vi "HandleObservationSync_002.vi"(8 "error in (no error)":errorcluster, 11 "S4GUI in":refnum<class "S4GUI.lvclass">) -> (0 "error out":errorcluster, 3 "S4GUI out":refnum<class "S4GUI.lvclass">)   [LabVIEW 2018, in "S4GUI.lvclass"] (continued)
          n221 = call "Read Instrument.lvclass.vi"("error in (no error)"=w570, "S4ACS_GUI in"=w571) -> ("error out"=w541:errorcluster, "Instrument.lvclass"=w542:refnum<class "Instrument.lvclass">, "S4ACS_GUI out"=w572:refnum<class "S4GUI.lvclass">)  [unwired: 7 in]
          n222 = disable-structure shown="Enabled" {
            disable-tunnel: w542 -> [w576 w589]
            disable-tunnel: w541 -> [w575 w588]
            disable-tunnel: [w574 w589] -> w540
            disable-tunnel: [w573 w588] -> w539
            frame Disabled {
              n223 = call "Read WPROT.vi"("error in (no error)"=w575, "Instrument in"=w576) -> ("error out"=w579:errorcluster, "Opt_Selector.lvclass"=w580:refnum<class "Opt_Selector.lvclass">, "Instrument out"=w586:refnum<class "Instrument.lvclass">)  [unwired: 7 in]
              n224 = call-dynamic "Read State Machine.vi"("error in (no error)"=w579, "Device in"=w580) -> ("error out"=w582:errorcluster, "State Machine.lvclass"=w584:refnum<class "State Machine.lvclass">, "Device out"=w581:refnum<class "Opt_Selector.lvclass">)  [unwired: 7 in]
              n225 = call "Next State.vi"("error in (no error)"=w582, "New_State"=30, "State Machine in"=w584) -> ("error out"=w578:errorcluster, "State Machine out"=w577:refnum<class "State Machine.lvclass">)  [unwired: 7 in]
              n226 = call-dynamic "Write State Machine.vi"("error in (no error)"=w578, "State Machine.lvclass"=w577, "Device in"=w581) -> ("error out"=w585:errorcluster, "Device out"=w587:refnum<class "Opt_Selector.lvclass">)  [unwired: 7 in]
              n227 = call "Write WPROT.vi"("error in (no error)"=w585, "Opt_Selector.lvclass"=w587, "Instrument in"=w586) -> ("error out"=w573:errorcluster, "Instrument out"=w574:refnum<class "Instrument.lvclass">)  [unwired: 7 in]
            }
            frame Enabled {
              # "depois do homing no WPSEL, o homing do WPROT é feito automaticamente pelo ICS"
            }
          }
          n228 = call "Read ASEL.vi"("error in (no error)"=w539, "Instrument in"=w540) -> ("error out"=w556:errorcluster, "Opt_Selector.lvclass"=w557:refnum<class "Opt_Selector.lvclass">, "Instrument out"=w563:refnum<class "Instrument.lvclass">)  [unwired: 7 in]
          n229 = call-dynamic "Read State Machine.vi"("error in (no error)"=w556, "Device in"=w557) -> ("error out"=w559:errorcluster, "State Machine.lvclass"=w561:refnum<class "State Machine.lvclass">, "Device out"=w558:refnum<class "Opt_Selector.lvclass">)  [unwired: 7 in]
          n230 = call "Next State.vi"("error in (no error)"=w559, "New_State"=30, "State Machine in"=w561) -> ("error out"=w555:errorcluster, "State Machine out"=w554:refnum<class "State Machine.lvclass">)  [unwired: 7 in]
          n231 = call-dynamic "Write State Machine.vi"("error in (no error)"=w555, "State Machine.lvclass"=w554, "Device in"=w558) -> ("error out"=w562:errorcluster, "Device out"=w564:refnum<class "Opt_Selector.lvclass">)  [unwired: 7 in]
          n232 = Increment(x=w565) -> (x+1=w567:u32)
          n233 = call "Write ASEL.vi"("error in (no error)"=w562, "Opt_Selector.lvclass"=w564, "Instrument in"=w563) -> ("error out"=w537:errorcluster, "Instrument out"=w538:refnum<class "Instrument.lvclass">)  [unwired: 7 in]
          n234 = call "Read GMIR.vi"("error in (no error)"=w537, "Instrument in"=w538) -> ("error out"=w545:errorcluster, "Opt_Continuous.lvclass"=w546:refnum<class "Opt_Continuous.lvclass">, "Instrument out"=w552:refnum<class "Instrument.lvclass">)  [unwired: 7 in]
          n235 = call-dynamic "Read State Machine.vi"("error in (no error)"=w545, "Device in"=w546) -> ("error out"=w548:errorcluster, "State Machine.lvclass"=w550:refnum<class "State Machine.lvclass">, "Device out"=w547:refnum<class "Opt_Continuous.lvclass">)  [unwired: 7 in]
          n236 = call "Next State.vi"("error in (no error)"=w548, "New_State"=30, "State Machine in"=w550) -> ("error out"=w544:errorcluster, "State Machine out"=w543:refnum<class "State Machine.lvclass">)  [unwired: 7 in]
          n237 = call-dynamic "Write State Machine.vi"("error in (no error)"=w544, "State Machine.lvclass"=w543, "Device in"=w547) -> ("error out"=w551:errorcluster, "Device out"=w553:refnum<class "Opt_Continuous.lvclass">)  [unwired: 7 in]
          n238 = call "Write GMIR.vi"("error in (no error)"=w551, "Opt_Continuous.lvclass"=w553, "Instrument in"=w552) -> ("error out"=w536:errorcluster, "Instrument out"=w535:refnum<class "Instrument.lvclass">)  [unwired: 7 in]
          n239 = call "Write Instrument.lvclass.vi"("error in (no error)"=w536, "Instrument.lvclass"=w535, "S4ACS_GUI in"=w572) -> ("error out"=w569:errorcluster, "S4ACS_GUI out"=w568:refnum<class "S4GUI.lvclass">)  [unwired: 7 in]
          n240 = Bundle By Name(cluster=w568, "Obs_state"=w567) -> (w566:refnum<class "S4GUI.lvclass">)
        }
        frame 223 {
          # "Espera terminar o homing de WPROT,ASEL e GFOC\nantes de seguir para o próximo estado."
          n241 = call "Read Instrument.lvclass.vi"("error in (no error)"=w614, "S4ACS_GUI in"=w615) -> ("error out"=w600:errorcluster, "Instrument.lvclass"=w601:refnum<class "Instrument.lvclass">, "S4ACS_GUI out"=w609:refnum<class "S4GUI.lvclass">)  [unwired: 7 in]
          n242 = call "Read ASEL.vi"("error in (no error)"=w600, "Instrument in"=w601) -> ("error out"=w605:errorcluster, "Opt_Selector.lvclass"=w591:refnum<class "Opt_Selector.lvclass">)  [unwired: 7 in, 1 out]
          n243 = call "Read GMIR.vi"("error in (no error)"=w600, "Instrument in"=w601) -> ("error out"=w602:errorcluster, "Opt_Continuous.lvclass"=w590:refnum<class "Opt_Continuous.lvclass">)  [unwired: 7 in, 1 out]
          n244 = disable-structure shown="Enabled" {
            disable-tunnel: [w619 w625] -> w608
            disable-tunnel: w601 -> [w618 _]
            disable-tunnel: w600 -> [w617 w625]
            disable-tunnel: [w616 0 ("State")] -> w599
            frame Disabled {
              n245 = call "Read WPROT.vi"("error in (no error)"=w617, "Instrument in"=w618) -> ("error out"=w621:errorcluster, "Opt_Selector.lvclass"=w620:refnum<class "Opt_Selector.lvclass">)  [unwired: 7 in, 1 out]
              n246 = call-dynamic "Read State Machine.vi"("error in (no error)"=w621, "Device in"=w620) -> ("error out"=w622:errorcluster, "State Machine.lvclass"=w623:refnum<class "State Machine.lvclass">)  [unwired: 7 in, 1 out]
              n247 = call-dynamic "Read State.vi"("error in (no error)"=w622, "State Machine in"=w623) -> ("error out"=w619:errorcluster, "State"=w616:i32)  [unwired: 7 in, 1 out]
            }
            frame Enabled {
            }
          }
          n248 = call-dynamic "Read State Machine.vi"("error in (no error)"=w605, "Device in"=w591) -> ("error out"=w606:errorcluster, "State Machine.lvclass"=w607:refnum<class "State Machine.lvclass">)  [unwired: 7 in, 1 out]
          n249 = call-dynamic "Read State Machine.vi"("error in (no error)"=w602, "Device in"=w590) -> ("error out"=w603:errorcluster, "State Machine.lvclass"=w604:refnum<class "State Machine.lvclass">)  [unwired: 7 in, 1 out]
          n250 = Increment(x=w611) -> (x+1=w610:u32)
          n251 = call-dynamic "Read State.vi"("error in (no error)"=w606, "State Machine in"=w607) -> ("error out"=w594:errorcluster, "State"=w598:i32)  [unwired: 7 in, 1 out]
          n252 = call-dynamic "Read State.vi"("error in (no error)"=w603, "State Machine in"=w604) -> ("error out"=w593:errorcluster, "State"=w597:i32)  [unwired: 7 in, 1 out]
          n253 = Compound Arithmetic op=ADD(w599, w598, w597) -> (w596:i32)
          n254 = Equal To 0?(x=w596) -> (x = 0?=w595:bool)
          n255 = Merge Errors(w608, w594, w593) -> (w592:errorcluster)
          n256 = Select(t=w610, s=w595, f=w611) -> (s? t:f=w612:u32)
          n257 = Bundle By Name(cluster=w609, "Obs_state"=w612) -> (w613:refnum<class "S4GUI.lvclass">)
        }
        frame 224 {
          # "40 x 0.25 = 10s"
          # "40 x 0.25 = 10s"
          # "40 x 0.25 = 10s"
          # "Manda WPSEL para OFF, CALW para OFF e ASEL para OFF"
          n258 = call "Read Instrument.lvclass.vi"("error in (no error)"=w699, "S4ACS_GUI in"=w700) -> ("error out"=w685:errorcluster, "Instrument.lvclass"=w686:refnum<class "Instrument.lvclass">, "S4ACS_GUI out"=w701:refnum<class "S4GUI.lvclass">)  [unwired: 7 in]
          n259 = call "Read WPSEL.vi"("error in (no error)"=w685, "Instrument in"=w686) -> ("error out"=w681:errorcluster, "Opt_Selector.lvclass"=w680:refnum<class "Opt_Selector.lvclass">, "Instrument out"=w693:refnum<class "Instrument.lvclass">)  [unwired: 7 in]
          n260 = call "Write target.vi"("error in (no error)"=w681, "target"=80.0, "Optics in"=w680) -> ("error out"=w684:errorcluster, "Optics out"=w679:refnum<class "Opt_Selector.lvclass">)  [unwired: 7 in]
          n261 = call "Write target name.vi"("error in (no error)"=w684, "target name"="OFF", "Optics in"=w679) -> ("error out"=w677:errorcluster, "Optics out"=w678:refnum<class "Opt_Selector.lvclass">)  [unwired: 7 in]
          n262 = call-dynamic "Read State Machine.vi"("error in (no error)"=w677, "Device in"=w678) -> ("error out"=w688:errorcluster, "State Machine.lvclass"=w690:refnum<class "State Machine.lvclass">, "Device out"=w687:refnum<class "Opt_Selector.lvclass">)  [unwired: 7 in]
          n263 = call "Next State.vi"("error in (no error)"=w688, "New_State"=1, "State Machine in"=w690) -> ("error out"=w638:errorcluster, "State Machine out"=w640:refnum<class "State Machine.lvclass">)  [unwired: 7 in]
          n264 = call-dynamic "Write Timer.vi"("error in (no error)"=w638, "Timer"=u32 40, "State Machine in"=w640) -> ("error out"=w637:errorcluster, "State Machine out"=w639:refnum<class "State Machine.lvclass">)  [unwired: 7 in]
          n265 = call-dynamic "Write State Machine.vi"("error in (no error)"=w637, "State Machine.lvclass"=w639, "Device in"=w687) -> ("error out"=w692:errorcluster, "Device out"=w694:refnum<class "Opt_Selector.lvclass">)  [unwired: 7 in]
          n266 = Increment(x=w691) -> (x+1=w696:u32)
          n267 = call "Write WPSEL.vi"("error in (no error)"=w692, "Opt_Selector.lvclass"=w694, "Instrument in"=w693) -> ("error out"=w652:errorcluster, "Instrument out"=w651:refnum<class "Instrument.lvclass">)  [unwired: 7 in]
          n268 = call "Read CALW.vi"("error in (no error)"=w652, "Instrument in"=w651) -> ("error out"=w668:errorcluster, "Opt_Selector.lvclass"=w650:refnum<class "Opt_Selector.lvclass">, "Instrument out"=w648:refnum<class "Instrument.lvclass">)  [unwired: 7 in]
          n269 = call "Write target.vi"("error in (no error)"=w668, "target"=0.0, "Optics in"=w650) -> ("error out"=w671:errorcluster, "Optics out"=w667:refnum<class "Opt_Selector.lvclass">)  [unwired: 7 in]
          n270 = call "Write target name.vi"("error in (no error)"=w671, "target name"="OFF", "Optics in"=w667) -> ("error out"=w665:errorcluster, "Optics out"=w666:refnum<class "Opt_Selector.lvclass">)  [unwired: 7 in]
          n271 = call-dynamic "Read State Machine.vi"("error in (no error)"=w665, "Device in"=w666) -> ("error out"=w673:errorcluster, "State Machine.lvclass"=w675:refnum<class "State Machine.lvclass">, "Device out"=w672:refnum<class "Opt_Selector.lvclass">)  [unwired: 7 in]
          n272 = call "Next State.vi"("error in (no error)"=w673, "New_State"=1, "State Machine in"=w675) -> ("error out"=w634:errorcluster, "State Machine out"=w635:refnum<class "State Machine.lvclass">)  [unwired: 7 in]
          n273 = call-dynamic "Write Timer.vi"("error in (no error)"=w634, "Timer"=u32 40, "State Machine in"=w635) -> ("error out"=w633:errorcluster, "State Machine out"=w632:refnum<class "State Machine.lvclass">)  [unwired: 7 in]
          n274 = call-dynamic "Write State Machine.vi"("error in (no error)"=w633, "State Machine.lvclass"=w632, "Device in"=w672) -> ("error out"=w676:errorcluster, "Device out"=w649:refnum<class "Opt_Selector.lvclass">)  [unwired: 7 in]
          n275 = call "Write CALW.vi"("error in (no error)"=w676, "Opt_Selector.lvclass"=w649, "Instrument in"=w648) -> ("error out"=w647:errorcluster, "Instrument out"=w646:refnum<class "Instrument.lvclass">)  [unwired: 7 in]
          n276 = call "Read ASEL.vi"("error in (no error)"=w647, "Instrument in"=w646) -> ("error out"=w656:errorcluster, "Opt_Selector.lvclass"=w645:refnum<class "Opt_Selector.lvclass">, "Instrument out"=w643:refnum<class "Instrument.lvclass">)  [unwired: 7 in]
          n277 = call "Write target.vi"("error in (no error)"=w656, "target"=0.0, "Optics in"=w645) -> ("error out"=w659:errorcluster, "Optics out"=w655:refnum<class "Opt_Selector.lvclass">)  [unwired: 7 in]
          n278 = call "Write target name.vi"("error in (no error)"=w659, "target name"="OFF", "Optics in"=w655) -> ("error out"=w653:errorcluster, "Optics out"=w654:refnum<class "Opt_Selector.lvclass">)  [unwired: 7 in]
          n279 = call-dynamic "Read State Machine.vi"("error in (no error)"=w653, "Device in"=w654) -> ("error out"=w661:errorcluster, "State Machine.lvclass"=w663:refnum<class "State Machine.lvclass">, "Device out"=w660:refnum<class "Opt_Selector.lvclass">)  [unwired: 7 in]
          n280 = call "Next State.vi"("error in (no error)"=w661, "New_State"=1, "State Machine in"=w663) -> ("error out"=w628:errorcluster, "State Machine out"=w629:refnum<class "State Machine.lvclass">)  [unwired: 7 in]
          n281 = call-dynamic "Write Timer.vi"("error in (no error)"=w628, "Timer"=u32 40, "State Machine in"=w629) -> ("error out"=w627:errorcluster, "State Machine out"=w626:refnum<class "State Machine.lvclass">)  [unwired: 7 in]
          n282 = call-dynamic "Write State Machine.vi"("error in (no error)"=w627, "State Machine.lvclass"=w626, "Device in"=w660) -> ("error out"=w664:errorcluster, "Device out"=w644:refnum<class "Opt_Selector.lvclass">)  [unwired: 7 in]
          n283 = call "Write ASEL.vi"("error in (no error)"=w664, "Opt_Selector.lvclass"=w644, "Instrument in"=w643) -> ("error out"=w641:errorcluster, "Instrument out"=w642:refnum<class "Instrument.lvclass">)  [unwired: 7 in]
          n284 = call "Write Instrument.lvclass.vi"("error in (no error)"=w641, "Instrument.lvclass"=w642, "S4ACS_GUI in"=w701) -> ("error out"=w698:errorcluster, "S4ACS_GUI out"=w697:refnum<class "S4GUI.lvclass">)  [unwired: 7 in]
          n285 = Bundle By Name(cluster=w697, "Obs_state"=w696) -> (w695:refnum<class "S4GUI.lvclass">)
        }
        frame 225 {
          # "Espera terminar o movimento de WPSEL, ASEL e CALW para CLEAR."
          n286 = call "Read Instrument.lvclass.vi"("error in (no error)"=w730, "S4ACS_GUI in"=w731) -> ("error out"=w713:errorcluster, "Instrument.lvclass"=w714:refnum<class "Instrument.lvclass">, "S4ACS_GUI out"=w722:refnum<class "S4GUI.lvclass">)  [unwired: 7 in]
          n287 = call "Read ASEL.vi"("error in (no error)"=w713, "Instrument in"=w714) -> ("error out"=w718:errorcluster, "Opt_Selector.lvclass"=w704:refnum<class "Opt_Selector.lvclass">)  [unwired: 7 in, 1 out]
          n288 = call "Read CALW.vi"("error in (no error)"=w713, "Instrument in"=w714) -> ("error out"=w715:errorcluster, "Opt_Selector.lvclass"=w703:refnum<class "Opt_Selector.lvclass">)  [unwired: 7 in, 1 out]
          n289 = call "Read WPSEL.vi"("error in (no error)"=w713, "Instrument in"=w714) -> ("error out"=w727:errorcluster, "Opt_Selector.lvclass"=w726:refnum<class "Opt_Selector.lvclass">)  [unwired: 7 in, 1 out]
          n290 = call-dynamic "Read State Machine.vi"("error in (no error)"=w715, "Device in"=w703) -> ("error out"=w716:errorcluster, "State Machine.lvclass"=w717:refnum<class "State Machine.lvclass">)  [unwired: 7 in, 1 out]
          n291 = call-dynamic "Read State Machine.vi"("error in (no error)"=w718, "Device in"=w704) -> ("error out"=w719:errorcluster, "State Machine.lvclass"=w720:refnum<class "State Machine.lvclass">)  [unwired: 7 in, 1 out]
          n292 = call-dynamic "Read State Machine.vi"("error in (no error)"=w727, "Device in"=w726) -> ("error out"=w728:errorcluster, "State Machine.lvclass"=w729:refnum<class "State Machine.lvclass">)  [unwired: 7 in, 1 out]
          n293 = call-dynamic "Read State.vi"("error in (no error)"=w719, "State Machine in"=w720) -> ("error out"=w707:errorcluster, "State"=w711:i32)  [unwired: 7 in, 1 out]
          n294 = call-dynamic "Read State.vi"("error in (no error)"=w716, "State Machine in"=w717) -> ("error out"=w706:errorcluster, "State"=w710:i32)  [unwired: 7 in, 1 out]
          n295 = call-dynamic "Read State.vi"("error in (no error)"=w728, "State Machine in"=w729) -> ("error out"=w721:errorcluster, "State"=w712:i32)  [unwired: 7 in, 1 out]
          n296 = Compound Arithmetic op=ADD(w712, w711, w710) -> (w709:i32)
          n297 = Equal To 0?(x=w709) -> (x = 0?=w708:bool)
          n298 = Merge Errors(w721, w707, w706) -> (w705:errorcluster)
          n299 = Select(t=u32 0, s=w708, f=w723) -> (s? t:f=w724:u32)
          n300 = Bundle By Name(cluster=w722, "Obs_state"=w724) -> (w725:refnum<class "S4GUI.lvclass">)
        }
        frame 230 {
          # "PARK:\nWPSEL = OFF\n(WPROT=NA)\nCALW=SHUTTER\nASEL=OFF"
          n301 = call "Read Instrument.lvclass.vi"("error in (no error)"=w799, "S4ACS_GUI in"=w800) -> ("error out"=w792:errorcluster, "Instrument.lvclass"=w793:refnum<class "Instrument.lvclass">, "S4ACS_GUI out"=w734:refnum<class "S4GUI.lvclass">)  [unwired: 7 in]
          n302 = call "Read WPSEL.vi"("error in (no error)"=w792, "Instrument in"=w793) -> ("error out"=w755:errorcluster, "Opt_Selector.lvclass"=w758:refnum<class "Opt_Selector.lvclass">, "Instrument out"=w788:refnum<class "Instrument.lvclass">)  [unwired: 7 in]
          n303 = call "Write target name.vi"("error in (no error)"=w755, "target name"="OFF", "Optics in"=w758) -> ("error out"=w754:errorcluster, "Optics out"=w757:refnum<class "Opt_Selector.lvclass">)  [unwired: 7 in]
          n304 = call "Write target.vi"("error in (no error)"=w754, "target"=80.0, "Optics in"=w757) -> ("error out"=w753:errorcluster, "Optics out"=w756:refnum<class "Opt_Selector.lvclass">)  [unwired: 7 in]
          n305 = call-dynamic "Read State Machine.vi"("error in (no error)"=w753, "Device in"=w756) -> ("error out"=w784:errorcluster, "State Machine.lvclass"=w786:refnum<class "State Machine.lvclass">, "Device out"=w783:refnum<class "Opt_Selector.lvclass">)  [unwired: 7 in]
          n306 = call "Next State.vi"("error in (no error)"=w784, "New_State"=1, "State Machine in"=w786) -> ("error out"=w763:errorcluster, "State Machine out"=w764:refnum<class "State Machine.lvclass">)  [unwired: 7 in]
          n307 = call-dynamic "Write State Machine.vi"("error in (no error)"=w763, "State Machine.lvclass"=w764, "Device in"=w783) -> ("error out"=w787:errorcluster, "Device out"=w789:refnum<class "Opt_Selector.lvclass">)  [unwired: 7 in]
          n308 = Increment(x=w794) -> (x+1=w796:u32)
          n309 = call "Write WPSEL.vi"("error in (no error)"=w787, "Opt_Selector.lvclass"=w789, "Instrument in"=w788) -> ("error out"=w767:errorcluster, "Instrument out"=w768:refnum<class "Instrument.lvclass">)  [unwired: 7 in]
          n310 = call "Read CALW.vi"("error in (no error)"=w767, "Instrument in"=w768) -> ("error out"=w747:errorcluster, "Opt_Selector.lvclass"=w746:refnum<class "Opt_Selector.lvclass">, "Instrument out"=w781:refnum<class "Instrument.lvclass">)  [unwired: 7 in]
          n311 = call "Write target name.vi"("error in (no error)"=w747, "target name"="SHUTTER", "Optics in"=w746) -> ("error out"=w750:errorcluster, "Optics out"=w745:refnum<class "Opt_Selector.lvclass">)  [unwired: 7 in]
          n312 = call "Write target.vi"("error in (no error)"=w750, "target"=216.0, "Optics in"=w745) -> ("error out"=w743:errorcluster, "Optics out"=w744:refnum<class "Opt_Selector.lvclass">)  [unwired: 7 in]
          n313 = call-dynamic "Read State Machine.vi"("error in (no error)"=w743, "Device in"=w744) -> ("error out"=w777:errorcluster, "State Machine.lvclass"=w779:refnum<class "State Machine.lvclass">, "Device out"=w776:refnum<class "Opt_Selector.lvclass">)  [unwired: 7 in]
          n314 = call "Next State.vi"("error in (no error)"=w777, "New_State"=1, "State Machine in"=w779) -> ("error out"=w761:errorcluster, "State Machine out"=w762:refnum<class "State Machine.lvclass">)  [unwired: 7 in]
          n315 = call-dynamic "Write State Machine.vi"("error in (no error)"=w761, "State Machine.lvclass"=w762, "Device in"=w776) -> ("error out"=w780:errorcluster, "Device out"=w782:refnum<class "Opt_Selector.lvclass">)  [unwired: 7 in]
          n316 = call "Write CALW.vi"("error in (no error)"=w780, "Opt_Selector.lvclass"=w782, "Instrument in"=w781) -> ("error out"=w765:errorcluster, "Instrument out"=w766:refnum<class "Instrument.lvclass">)  [unwired: 7 in]
          n317 = call "Read ASEL.vi"("error in (no error)"=w765, "Instrument in"=w766) -> ("error out"=w736:errorcluster, "Opt_Selector.lvclass"=w739:refnum<class "Opt_Selector.lvclass">, "Instrument out"=w774:refnum<class "Instrument.lvclass">)  [unwired: 7 in]
          n318 = call "Write target name.vi"("error in (no error)"=w736, "target name"="OFF", "Optics in"=w739) -> ("error out"=w742:errorcluster, "Optics out"=w738:refnum<class "Opt_Selector.lvclass">)  [unwired: 7 in]
          n319 = call "Write target.vi"("error in (no error)"=w742, "target"=0.0, "Optics in"=w738) -> ("error out"=w735:errorcluster, "Optics out"=w737:refnum<class "Opt_Selector.lvclass">)  [unwired: 7 in]
          n320 = call-dynamic "Read State Machine.vi"("error in (no error)"=w735, "Device in"=w737) -> ("error out"=w770:errorcluster, "State Machine.lvclass"=w772:refnum<class "State Machine.lvclass">, "Device out"=w769:refnum<class "Opt_Selector.lvclass">)  [unwired: 7 in]
          n321 = call "Next State.vi"("error in (no error)"=w770, "New_State"=1, "State Machine in"=w772) -> ("error out"=w759:errorcluster, "State Machine out"=w760:refnum<class "State Machine.lvclass">)  [unwired: 7 in]
          n322 = call-dynamic "Write State Machine.vi"("error in (no error)"=w759, "State Machine.lvclass"=w760, "Device in"=w769) -> ("error out"=w773:errorcluster, "Device out"=w775:refnum<class "Opt_Selector.lvclass">)  [unwired: 7 in]
          n323 = call "Write ASEL.vi"("error in (no error)"=w773, "Opt_Selector.lvclass"=w775, "Instrument in"=w774) -> ("error out"=w791:errorcluster, "Instrument out"=w790:refnum<class "Instrument.lvclass">)  [unwired: 7 in]
          n324 = Bundle By Name(cluster=w734, "Error Msg"="Parking in progress. Wait....") -> (w733:refnum<class "S4GUI.lvclass">)
          n325 = call "Write Instrument.lvclass.vi"("error in (no error)"=w791, "Instrument.lvclass"=w790, "S4ACS_GUI in"=w733) -> ("error out"=w798:errorcluster, "S4ACS_GUI out"=w797:refnum<class "S4GUI.lvclass">)  [unwired: 7 in]
          n326 = Bundle By Name(cluster=w797, "Obs_state"=w796) -> (w795:refnum<class "S4GUI.lvclass">)
        }
        frame 231 {
          # "Espera terminar o parking de WPSEL,CALW e ASEL\nantes de encerrar aplicacao (exit=True)."
          n327 = call "Read Instrument.lvclass.vi"("error in (no error)"=w829, "S4ACS_GUI in"=w830) -> ("error out"=w811:errorcluster, "Instrument.lvclass"=w812:refnum<class "Instrument.lvclass">, "S4ACS_GUI out"=w820:refnum<class "S4GUI.lvclass">)  [unwired: 7 in]
          n328 = call "Read CALW.vi"("error in (no error)"=w811, "Instrument in"=w812) -> ("error out"=w816:errorcluster, "Opt_Selector.lvclass"=w802:refnum<class "Opt_Selector.lvclass">)  [unwired: 7 in, 1 out]
          n329 = call "Read ASEL.vi"("error in (no error)"=w811, "Instrument in"=w812) -> ("error out"=w813:errorcluster, "Opt_Selector.lvclass"=w801:refnum<class "Opt_Selector.lvclass">)  [unwired: 7 in, 1 out]
          n330 = call "Read WPSEL.vi"("error in (no error)"=w811, "Instrument in"=w812) -> ("error out"=w826:errorcluster, "Opt_Selector.lvclass"=w825:refnum<class "Opt_Selector.lvclass">)  [unwired: 7 in, 1 out]
          n331 = call-dynamic "Read State Machine.vi"("error in (no error)"=w816, "Device in"=w802) -> ("error out"=w817:errorcluster, "State Machine.lvclass"=w818:refnum<class "State Machine.lvclass">)  [unwired: 7 in, 1 out]
          n332 = call-dynamic "Read State Machine.vi"("error in (no error)"=w813, "Device in"=w801) -> ("error out"=w814:errorcluster, "State Machine.lvclass"=w815:refnum<class "State Machine.lvclass">)  [unwired: 7 in, 1 out]
          n333 = call-dynamic "Read State Machine.vi"("error in (no error)"=w826, "Device in"=w825) -> ("error out"=w827:errorcluster, "State Machine.lvclass"=w828:refnum<class "State Machine.lvclass">)  [unwired: 7 in, 1 out]
          n334 = Increment(x=w822) -> (x+1=w821:u32)
          n335 = call-dynamic "Read State.vi"("error in (no error)"=w817, "State Machine in"=w818) -> ("error out"=w805:errorcluster, "State"=w809:i32)  [unwired: 7 in, 1 out]
          n336 = call-dynamic "Read State.vi"("error in (no error)"=w814, "State Machine in"=w815) -> ("error out"=w804:errorcluster, "State"=w808:i32)  [unwired: 7 in, 1 out]
          n337 = call-dynamic "Read State.vi"("error in (no error)"=w827, "State Machine in"=w828) -> ("error out"=w819:errorcluster, "State"=w810:i32)  [unwired: 7 in, 1 out]
          n338 = Compound Arithmetic op=ADD(w810, w809, w808) -> (w807:i32)
          n339 = Equal To 0?(x=w807) -> (x = 0?=w806:bool)
          n340 = Merge Errors(w819, w805, w804) -> (w803:errorcluster)
          n341 = Select(t=w821, s=w806, f=w822) -> (s? t:f=w823:u32)
          n342 = Bundle By Name(cluster=w820, "Obs_state"=w823) -> (w824:refnum<class "S4GUI.lvclass">)
        }
        frame 232 {
          n343 = Increment(x=w832) -> (x+1=w831:u32)
          n344 = Tick Count (ms)() -> (millisecond timer value=w833:u32)
          n345 = local write "time1"(w833) -> ()
          n346 = Bundle By Name(cluster=w836, "Obs_state"=w831) -> (w834:refnum<class "S4GUI.lvclass">)
        }
        frame 233 {
          # "Aguarda 1s para atualização do painel da GUI antes de encerrar..."
          n347 = local read "time1"() -> (w840:u32)
          n348 = Tick Count (ms)() -> (millisecond timer value=w841:u32)
          n349 = Subtract(x=w841, y=w840) -> (x-y=w839:u32)
          n350 = Greater?(x=w839, y=u32 1000) -> (0:w837:bool)
          n351 = case shown="True" w837 {
            tunnel: w843 -> [w847 w849]
            tunnel: [w847 w848] -> w842
            frame False {
            }
            frame True {
              n352 = Increment(x=w849) -> (x+1=w848:u32)
            }
          }
          n353 = Bundle By Name(cluster=w846, "Obs_state"=w842) -> (w844:refnum<class "S4GUI.lvclass">)
        }
        frame 234 {
          n354 = Bundle By Name(cluster=w854, "Obs_state"=u32 0, "exit"=TRUE) -> (w852:refnum<class "S4GUI.lvclass">)
        }
        frame 251 {
          n355 = flat-sequence {
            tunnel: w903 -> [w1058]
            tunnel: [w1058] -> w902
            frame #0 {
              n356 = Tick Count (ms)() -> (millisecond timer value=→"time3":u32)
            }
          }
          n357 = call-dynamic "Read AcquisitionA.vi"("error in (no error)"=w902, "S4ACS_GUI in"=w920) -> ("error out"=w887:errorcluster, "Acquisition.lvclass"=w885:refnum<class "Acquisition.lvclass">, "S4ACS_GUI out"=w922:refnum<class "S4GUI.lvclass">)  [unwired: 7 in]
          n358 = call-dynamic "Read enabled.vi"("error in (no error)"=w887, "Server in"=w885) -> ("error out"=w886:errorcluster, "enabled"=w882:bool, "Server out"=w884:refnum<class "Acquisition.lvclass">)  [unwired: 7 in]
          n359 = call "Read connection.vi"("error in (no error)"=w886, "Server in"=w884) -> ("error out"=w918:errorcluster, "connection"=w888:bool, "Server out"=w917:refnum<class "Acquisition.lvclass">)  [unwired: 7 in]
          n360 = And(x=w888, y=w882) -> (x .and. y?=w883:bool)
          n361 = case shown="True" w883 {
            tunnel: [w1038 w1057] -> w923
            tunnel: [w1037 w1056] -> w921
            tunnel: w918 -> [w1037 w1055]
            tunnel: w917 -> [w1038 w1054]
            tunnel: w882 -> [w1034 _]
            tunnel: [w1033 u32 0] -> w881
            frame False {
              n362 = Select(t=u32 1, s=w1034, f=u32 0) -> (s? t:f=w1033:u32)
            }
            frame True {
              # "configura o canal,\nmas não dispara\na exposicao."
              n363 = call-dynamic "Read Channel.vi"("error in (no error)"=w1055, "Acquisition in"=w1054) -> ("error out"=w1044:errorcluster, "Channel.lvclass"=w1046:refnum<class "Channel.lvclass">, "Acquisition out"=w1053:refnum<class "Acquisition.lvclass">)  [unwired: 7 in]
              n364 = call-dynamic "Write expose.vi"("error in (no error)"=w1044, "expose"=FALSE, "Channel in"=w1046) -> ("error out"=w1043:errorcluster, "Channel out"=w1045:refnum<class "Channel.lvclass">)  [unwired: 7 in]
              n365 = call-dynamic "Read State Machine.vi"("error in (no error)"=w1043, "Device in"=w1045) -> ("error out"=w1050:errorcluster, "State Machine.lvclass"=w1052:refnum<class "State Machine.lvclass">, "Device out"=w1048:refnum<class "Channel.lvclass">)  [unwired: 7 in]
              n366 = call "Next State.vi"("error in (no error)"=w1050, "New_State"=1, "State Machine in"=w1052) -> ("error out"=w1040:errorcluster, "State Machine out"=w1041:refnum<class "State Machine.lvclass">)  [unwired: 7 in]
              n367 = call-dynamic "Write State Machine.vi"("error in (no error)"=w1040, "State Machine.lvclass"=w1041, "Device in"=w1048) -> ("error out"=w1047:errorcluster, "Device out"=w1049:refnum<class "Channel.lvclass">)  [unwired: 7 in]
              n368 = call-dynamic "Write Channel.vi"("error in (no error)"=w1047, "Channel.lvclass"=w1049, "Acquisition in"=w1053) -> ("error out"=w1056:errorcluster, "Acquisition out"=w1057:refnum<class "Acquisition.lvclass">)  [unwired: 7 in]
            }
          }
          n369 = call-dynamic "Write AcquisitionA.vi"("error in (no error)"=w921, "Acquisition.lvclass"=w923, "S4ACS_GUI in"=w922) -> ("error out"=w913:errorcluster, "S4ACS_GUI out"=w912:refnum<class "S4GUI.lvclass">)  [unwired: 7 in]
          n370 = call "Read AcquisitionB.vi"("error in (no error)"=w913, "S4ACS_GUI in"=w912) -> ("error out"=w871:errorcluster, "Acquisition.lvclass"=w873:refnum<class "Acquisition.lvclass">, "S4ACS_GUI out"=w914:refnum<class "S4GUI.lvclass">)  [unwired: 7 in]
          n371 = call-dynamic "Read enabled.vi"("error in (no error)"=w871, "Server in"=w873) -> ("error out"=w870:errorcluster, "enabled"=w855:bool, "Server out"=w872:refnum<class "Acquisition.lvclass">)  [unwired: 7 in]
          n372 = call "Read connection.vi"("error in (no error)"=w870, "Server in"=w872) -> ("error out"=w899:errorcluster, "connection"=w874:bool, "Server out"=w900:refnum<class "Acquisition.lvclass">)  [unwired: 7 in]
          n373 = And(x=w874, y=w855) -> (x .and. y?=w875:bool)
          n374 = case shown="True" w875 {
            tunnel: [w1013 w1032] -> w898
            tunnel: [w1012 w1031] -> w897
            tunnel: w899 -> [w1012 w1030]
            tunnel: w900 -> [w1013 w1029]
            tunnel: [w1009 u32 0 ("f")] -> w878
            tunnel: w855 -> [w1008 _]
            frame False {
              n375 = Select(t=u32 2, s=w1008, f=u32 0) -> (s? t:f=w1009:u32)
            }
            frame True {
              # "configura o canal,\nmas não dispara\na exposicao."
              n376 = call-dynamic "Read Channel.vi"("error in (no error)"=w1030, "Acquisition in"=w1029) -> ("error out"=w1019:errorcluster, "Channel.lvclass"=w1021:refnum<class "Channel.lvclass">, "Acquisition out"=w1028:refnum<class "Acquisition.lvclass">)  [unwired: 7 in]
              n377 = call-dynamic "Write expose.vi"("error in (no error)"=w1019, "expose"=FALSE, "Channel in"=w1021) -> ("error out"=w1018:errorcluster, "Channel out"=w1020:refnum<class "Channel.lvclass">)  [unwired: 7 in]
              n378 = call-dynamic "Read State Machine.vi"("error in (no error)"=w1018, "Device in"=w1020) -> ("error out"=w1025:errorcluster, "State Machine.lvclass"=w1027:refnum<class "State Machine.lvclass">, "Device out"=w1023:refnum<class "Channel.lvclass">)  [unwired: 7 in]
              n379 = call "Next State.vi"("error in (no error)"=w1025, "New_State"=1, "State Machine in"=w1027) -> ("error out"=w1015:errorcluster, "State Machine out"=w1016:refnum<class "State Machine.lvclass">)  [unwired: 7 in]
              n380 = call-dynamic "Write State Machine.vi"("error in (no error)"=w1015, "State Machine.lvclass"=w1016, "Device in"=w1023) -> ("error out"=w1022:errorcluster, "Device out"=w1024:refnum<class "Channel.lvclass">)  [unwired: 7 in]
              n381 = call-dynamic "Write Channel.vi"("error in (no error)"=w1022, "Channel.lvclass"=w1024, "Acquisition in"=w1028) -> ("error out"=w1031:errorcluster, "Acquisition out"=w1032:refnum<class "Acquisition.lvclass">)  [unwired: 7 in]
            }
          }
          n382 = call "Write AcquisitionB.vi"("error in (no error)"=w897, "Acquisition.lvclass"=w898, "S4ACS_GUI in"=w914) -> ("error out"=w909:errorcluster, "S4ACS_GUI out"=w908:refnum<class "S4GUI.lvclass">)  [unwired: 7 in]
          n383 = call-dynamic "Read AcquisitionC.vi"("error in (no error)"=w909, "S4ACS_GUI in"=w908) -> ("error out"=w867:errorcluster, "Acquisition.lvclass"=w869:refnum<class "Acquisition.lvclass">, "S4ACS_GUI out"=w911:refnum<class "S4GUI.lvclass">)  [unwired: 7 in]
          n384 = call-dynamic "Read enabled.vi"("error in (no error)"=w867, "Server in"=w869) -> ("error out"=w866:errorcluster, "enabled"=w856:bool, "Server out"=w868:refnum<class "Acquisition.lvclass">)  [unwired: 7 in]
          n385 = call "Read connection.vi"("error in (no error)"=w866, "Server in"=w868) -> ("error out"=w895:errorcluster, "connection"=w865:bool, "Server out"=w896:refnum<class "Acquisition.lvclass">)  [unwired: 7 in]
          n386 = And(x=w865, y=w856) -> (x .and. y?=w864:bool)
          n387 = case shown="True" w864 {
            tunnel: [w988 w1007] -> w894
            tunnel: [w987 w1006] -> w893
            tunnel: w895 -> [w987 w1005]
            tunnel: w896 -> [w988 w1004]
            tunnel: [w984 u32 0 ("f")] -> w877
            tunnel: w856 -> [w983 _]
            frame False {
              n388 = Select(t=u32 4, s=w983, f=u32 0) -> (s? t:f=w984:u32)
            }
            frame True {
              # "configura o canal,\nmas não dispara\na exposicao."
              n389 = call-dynamic "Read Channel.vi"("error in (no error)"=w1005, "Acquisition in"=w1004) -> ("error out"=w994:errorcluster, "Channel.lvclass"=w996:refnum<class "Channel.lvclass">, "Acquisition out"=w1003:refnum<class "Acquisition.lvclass">)  [unwired: 7 in]
              n390 = call-dynamic "Write expose.vi"("error in (no error)"=w994, "expose"=FALSE, "Channel in"=w996) -> ("error out"=w993:errorcluster, "Channel out"=w995:refnum<class "Channel.lvclass">)  [unwired: 7 in]
              n391 = call-dynamic "Read State Machine.vi"("error in (no error)"=w993, "Device in"=w995) -> ("error out"=w1000:errorcluster, "State Machine.lvclass"=w1002:refnum<class "State Machine.lvclass">, "Device out"=w998:refnum<class "Channel.lvclass">)  [unwired: 7 in]
              n392 = call "Next State.vi"("error in (no error)"=w1000, "New_State"=1, "State Machine in"=w1002) -> ("error out"=w990:errorcluster, "State Machine out"=w991:refnum<class "State Machine.lvclass">)  [unwired: 7 in]
              n393 = call-dynamic "Write State Machine.vi"("error in (no error)"=w990, "State Machine.lvclass"=w991, "Device in"=w998) -> ("error out"=w997:errorcluster, "Device out"=w999:refnum<class "Channel.lvclass">)  [unwired: 7 in]
              n394 = call-dynamic "Write Channel.vi"("error in (no error)"=w997, "Channel.lvclass"=w999, "Acquisition in"=w1003) -> ("error out"=w1006:errorcluster, "Acquisition out"=w1007:refnum<class "Acquisition.lvclass">)  [unwired: 7 in]
            }
          }
          n395 = call-dynamic "Write AcquisitionC.vi"("error in (no error)"=w893, "Acquisition.lvclass"=w894, "S4ACS_GUI in"=w911) -> ("error out"=w907:errorcluster, "S4ACS_GUI out"=w906:refnum<class "S4GUI.lvclass">)  [unwired: 7 in]
          n396 = call-dynamic "Read AcquisitionD.vi"("error in (no error)"=w907, "S4ACS_GUI in"=w906) -> ("error out"=w861:errorcluster, "Acquisition.lvclass"=w863:refnum<class "Acquisition.lvclass">, "S4ACS_GUI out"=w910:refnum<class "S4GUI.lvclass">)  [unwired: 7 in]
          n397 = call-dynamic "Read enabled.vi"("error in (no error)"=w861, "Server in"=w863) -> ("error out"=w860:errorcluster, "enabled"=w857:bool, "Server out"=w862:refnum<class "Acquisition.lvclass">)  [unwired: 7 in]
          n398 = call "Read connection.vi"("error in (no error)"=w860, "Server in"=w862) -> ("error out"=w891:errorcluster, "connection"=w859:bool, "Server out"=w892:refnum<class "Acquisition.lvclass">)  [unwired: 7 in]
          n399 = And(x=w859, y=w857) -> (x .and. y?=w858:bool)
          n400 = case shown="True" w858 {
            tunnel: [w963 w982] -> w890
            tunnel: [w962 w981] -> w889
            tunnel: w891 -> [w962 w980]
            tunnel: w892 -> [w963 w979]
            tunnel: [w959 u32 0 ("f")] -> w876
            tunnel: w857 -> [w958 _]
            frame False {
              n401 = Select(t=u32 8, s=w958, f=u32 0) -> (s? t:f=w959:u32)
            }
            frame True {
              # "configura o canal,\nmas não dispara\na exposicao."
              n402 = call-dynamic "Read Channel.vi"("error in (no error)"=w980, "Acquisition in"=w979) -> ("error out"=w969:errorcluster, "Channel.lvclass"=w971:refnum<class "Channel.lvclass">, "Acquisition out"=w978:refnum<class "Acquisition.lvclass">)  [unwired: 7 in]
              n403 = call-dynamic "Write expose.vi"("error in (no error)"=w969, "expose"=FALSE, "Channel in"=w971) -> ("error out"=w968:errorcluster, "Channel out"=w970:refnum<class "Channel.lvclass">)  [unwired: 7 in]
              n404 = call-dynamic "Read State Machine.vi"("error in (no error)"=w968, "Device in"=w970) -> ("error out"=w975:errorcluster, "State Machine.lvclass"=w977:refnum<class "State Machine.lvclass">, "Device out"=w973:refnum<class "Channel.lvclass">)  [unwired: 7 in]
              n405 = call "Next State.vi"("error in (no error)"=w975, "New_State"=1, "State Machine in"=w977) -> ("error out"=w965:errorcluster, "State Machine out"=w966:refnum<class "State Machine.lvclass">)  [unwired: 7 in]
              n406 = call-dynamic "Write State Machine.vi"("error in (no error)"=w965, "State Machine.lvclass"=w966, "Device in"=w973) -> ("error out"=w972:errorcluster, "Device out"=w974:refnum<class "Channel.lvclass">)  [unwired: 7 in]
              n407 = call-dynamic "Write Channel.vi"("error in (no error)"=w972, "Channel.lvclass"=w974, "Acquisition in"=w978) -> ("error out"=w981:errorcluster, "Acquisition out"=w982:refnum<class "Acquisition.lvclass">)  [unwired: 7 in]
            }
          }
          n408 = call-dynamic "Write AcquisitionD.vi"("error in (no error)"=w889, "Acquisition.lvclass"=w890, "S4ACS_GUI in"=w910) -> ("error out"=w905:errorcluster, "S4ACS_GUI out"=w904:refnum<class "S4GUI.lvclass">)  [unwired: 7 in]
          n409 = Compound Arithmetic op=ADD(w881, w878, w877, w876) -> (w880:u32)
          n410 = case shown="0, Default" w880 {
            tunnel: w916 -> [w927 _ _ _ _ _ _ _ _ _ _ _ _ _ _ _]
            tunnel: [w926 u32 1 ("Obs_state") u32 1 ("Obs_state") u32 1 ("Obs_state") u32 1 ("Obs_state") u32 1 ("Obs_state") u32 1 ("Obs_state") u32 1 ("Obs_state") u32 1 ("Obs_state") u32 1 ("Obs_state") u32 1 ("Obs_state") u32 1 ("Obs_state") u32 1 ("Obs_state") u32 1 ("Obs_state") u32 1 ("Obs_state") u32 1 ("Obs_state")] -> w915
            tunnel: ["" ("Error Msg") "ERROR: Lost channel 1 connection... - HandleObservationSync.vi state 251" ("Error Msg") "ERROR: Lost channel 2 connection...- HandleObservationSync.vi state 251" ("Error Msg") "ERROR: Lost channels 1 and 2 connection...- HandleObservationSync.vi state 251" ("Error Msg") "ERROR: Lost channel 3 connection...- HandleObservationSync.vi state 251" ("Error Msg") "ERROR: Lost channels 1 and  3 connection...- HandleObservationSync.vi state 251" ("Error Msg") "ERROR:  Lost channels 2 and  3 connection...- HandleObservationSync.vi state 251" ("Error Msg") "ERROR:  Lost channels 1, 2 and  3 connection...- HandleObservationSync.vi state 251" ("Error Msg") "ERROR: Lost channel 4 connection...- HandleObservationSync.vi state 251" ("Error Msg") "ERROR:  Lost channels 1 and 4 connection...- HandleObservationSync.vi state 251" ("Error Msg") "ERROR:  Lost channels 2 and 4 connection...- HandleObservationSync.vi state 251" ("Error Msg") "ERROR: Lost channels 1, 2 and 4 connection...- HandleObservationSync.vi state 251" ("Error Msg") "ERROR: Lost channels 3 and 4 connection...- HandleObservationSync.vi state 251" ("Error Msg") "ERROR: Lost channels 1, 3 and 4 connection...- HandleObservationSync.vi state 251" ("Error Msg") "ERROR: Lost channels 2, 3 and 4 connection...- HandleObservationSync.vi state 251" ("Error Msg") "ERROR: Lost channels 1, 2, 3 and 4 connection...- HandleObservationSync.vi state 251" ("Error Msg")] -> w879
            frame 0, Default {
              n411 = Tick Count (ms)() -> (millisecond timer value=→"time307":u32)
              n412 = Increment(x=w927) -> (x+1=w926:u32)
            }
            frame 1 {
            }
            frame 2 {
            }
            frame 3 {
            }
            frame 4 {
            }
            frame 5 {
            }
            frame 6 {
            }
            frame 7 {
            }
            frame 8 {
            }
            frame 9 {
            }
            frame 10 {
            }
            frame 11 {
            }
            frame 12 {
            }
            frame 13 {
            }
            frame 14 {
            }
            frame 15 {
            }
          }
          n413 = Bundle By Name(cluster=w904, "Obs_state"=w915, "cyclesDone"=u32 0, "Error Msg"=w879) -> (w919:refnum<class "S4GUI.lvclass">)
        }
        frame 252 {
          w1081 = 38 ("x")
          w1084 = 28 ("x")
          # "Se algum canal foi pra 38: Texp inválido \npara a configuração do CCD."
          # "Se algum canal foi pra 28: ERRO na inicialização."
          # "Espera terminar a execução da preparação\ndos 4 canais antes de ir ao proximo passo \nda Observação."
          n414 = flat-sequence {
            tunnel: w1113 -> [w1250]
            tunnel: [w1250] -> w1112
            frame #0 {
              n415 = Tick Count (ms)() -> (millisecond timer value=→"time4":u32)
            }
          }
          n416 = call-dynamic "Read AcquisitionA.vi"("error in (no error)"=w1112, "S4ACS_GUI in"=w1122) -> ("error out"=w1110:errorcluster, "Acquisition.lvclass"=w1111:refnum<class "Acquisition.lvclass">, "S4ACS_GUI out"=w1124:refnum<class "S4GUI.lvclass">)  [unwired: 7 in]
          n417 = call "Read connection.vi"("error in (no error)"=w1110, "Server in"=w1111) -> ("error out"=w1108:errorcluster, "connection"=w1107:bool, "Server out"=w1109:refnum<class "Acquisition.lvclass">)  [unwired: 7 in]
          n418 = case shown="True" w1107 {
            tunnel: w1109 -> [w1233 w1249]
            tunnel: w1108 -> [w1232 w1248]
            tunnel: [w1233 w1246] -> w1125
            tunnel: [w1232 w1245] -> w1123
            tunnel: [0 ("State") w1235] -> w1080
            frame False {
            }
            frame True {
              n419 = call-dynamic "Read Channel.vi"("error in (no error)"=w1248, "Acquisition in"=w1249) -> ("error out"=w1244:errorcluster, "Channel.lvclass"=w1243:refnum<class "Channel.lvclass">, "Acquisition out"=w1247:refnum<class "Acquisition.lvclass">)  [unwired: 7 in]
              n420 = call-dynamic "Read State Machine.vi"("error in (no error)"=w1244, "Device in"=w1243) -> ("error out"=w1237:errorcluster, "State Machine.lvclass"=w1239:refnum<class "State Machine.lvclass">, "Device out"=w1241:refnum<class "Channel.lvclass">)  [unwired: 7 in]
              n421 = call-dynamic "Read State.vi"("error in (no error)"=w1237, "State Machine in"=w1239) -> ("error out"=w1236:errorcluster, "State"=w1235:i32, "State Machine out"=w1238:refnum<class "State Machine.lvclass">)  [unwired: 7 in]
              n422 = call-dynamic "Write State Machine.vi"("error in (no error)"=w1236, "State Machine.lvclass"=w1238, "Device in"=w1241) -> ("error out"=w1240:errorcluster, "Device out"=w1242:refnum<class "Channel.lvclass">)  [unwired: 7 in]
              n423 = call-dynamic "Write Channel.vi"("error in (no error)"=w1240, "Channel.lvclass"=w1242, "Acquisition in"=w1247) -> ("error out"=w1245:errorcluster, "Acquisition out"=w1246:refnum<class "Acquisition.lvclass">)  [unwired: 7 in]
            }
          }
          n424 = call-dynamic "Write AcquisitionA.vi"("error in (no error)"=w1123, "Acquisition.lvclass"=w1125, "S4ACS_GUI in"=w1124) -> ("error out"=w1119:errorcluster, "S4ACS_GUI out"=w1118:refnum<class "S4GUI.lvclass">)  [unwired: 7 in]
          n425 = call "Read AcquisitionB.vi"("error in (no error)"=w1119, "S4ACS_GUI in"=w1118) -> ("error out"=w1102:errorcluster, "Acquisition.lvclass"=w1105:refnum<class "Acquisition.lvclass">, "S4ACS_GUI out"=w1106:refnum<class "S4GUI.lvclass">)  [unwired: 7 in]
          n426 = call "Read connection.vi"("error in (no error)"=w1102, "Server in"=w1105) -> ("error out"=w1101:errorcluster, "connection"=w1103:bool, "Server out"=w1104:refnum<class "Acquisition.lvclass">)  [unwired: 7 in]
          n427 = case shown="True" w1103 {
            tunnel: w1104 -> [w1215 w1231]
            tunnel: w1101 -> [w1214 w1230]
            tunnel: [w1215 w1228] -> w1100
            tunnel: [w1214 w1227] -> w1099
            tunnel: [0 ("State") w1217] -> w1079
            frame False {
            }
            frame True {
              n428 = call-dynamic "Read Channel.vi"("error in (no error)"=w1230, "Acquisition in"=w1231) -> ("error out"=w1226:errorcluster, "Channel.lvclass"=w1225:refnum<class "Channel.lvclass">, "Acquisition out"=w1229:refnum<class "Acquisition.lvclass">)  [unwired: 7 in]
              n429 = call-dynamic "Read State Machine.vi"("error in (no error)"=w1226, "Device in"=w1225) -> ("error out"=w1219:errorcluster, "State Machine.lvclass"=w1221:refnum<class "State Machine.lvclass">, "Device out"=w1223:refnum<class "Channel.lvclass">)  [unwired: 7 in]
              n430 = call-dynamic "Read State.vi"("error in (no error)"=w1219, "State Machine in"=w1221) -> ("error out"=w1218:errorcluster, "State"=w1217:i32, "State Machine out"=w1220:refnum<class "State Machine.lvclass">)  [unwired: 7 in]
              n431 = call-dynamic "Write State Machine.vi"("error in (no error)"=w1218, "State Machine.lvclass"=w1220, "Device in"=w1223) -> ("error out"=w1222:errorcluster, "Device out"=w1224:refnum<class "Channel.lvclass">)  [unwired: 7 in]
              n432 = call-dynamic "Write Channel.vi"("error in (no error)"=w1222, "Channel.lvclass"=w1224, "Acquisition in"=w1229) -> ("error out"=w1227:errorcluster, "Acquisition out"=w1228:refnum<class "Acquisition.lvclass">)  [unwired: 7 in]
            }
          }
          n433 = call "Write AcquisitionB.vi"("error in (no error)"=w1099, "Acquisition.lvclass"=w1100, "S4ACS_GUI in"=w1106) -> ("error out"=w1117:errorcluster, "S4ACS_GUI out"=w1116:refnum<class "S4GUI.lvclass">)  [unwired: 7 in]
          n434 = call-dynamic "Read AcquisitionC.vi"("error in (no error)"=w1117, "S4ACS_GUI in"=w1116) -> ("error out"=w1097:errorcluster, "Acquisition.lvclass"=w1098:refnum<class "Acquisition.lvclass">, "S4ACS_GUI out"=w1121:refnum<class "S4GUI.lvclass">)  [unwired: 7 in]
          n435 = call "Read connection.vi"("error in (no error)"=w1097, "Server in"=w1098) -> ("error out"=w1096:errorcluster, "connection"=w1094:bool, "Server out"=w1095:refnum<class "Acquisition.lvclass">)  [unwired: 7 in]
          n436 = case shown="True" w1094 {
            tunnel: w1095 -> [w1197 w1213]
            tunnel: w1096 -> [w1196 w1212]
            tunnel: [w1197 w1210] -> w1093
            tunnel: [w1196 w1209] -> w1092
            tunnel: [0 ("State") w1199] -> w1078
            frame False {
            }
            frame True {
              n437 = call-dynamic "Read Channel.vi"("error in (no error)"=w1212, "Acquisition in"=w1213) -> ("error out"=w1208:errorcluster, "Channel.lvclass"=w1207:refnum<class "Channel.lvclass">, "Acquisition out"=w1211:refnum<class "Acquisition.lvclass">)  [unwired: 7 in]
              n438 = call-dynamic "Read State Machine.vi"("error in (no error)"=w1208, "Device in"=w1207) -> ("error out"=w1201:errorcluster, "State Machine.lvclass"=w1203:refnum<class "State Machine.lvclass">, "Device out"=w1205:refnum<class "Channel.lvclass">)  [unwired: 7 in]
              n439 = call-dynamic "Read State.vi"("error in (no error)"=w1201, "State Machine in"=w1203) -> ("error out"=w1200:errorcluster, "State"=w1199:i32, "State Machine out"=w1202:refnum<class "State Machine.lvclass">)  [unwired: 7 in]
              n440 = call-dynamic "Write State Machine.vi"("error in (no error)"=w1200, "State Machine.lvclass"=w1202, "Device in"=w1205) -> ("error out"=w1204:errorcluster, "Device out"=w1206:refnum<class "Channel.lvclass">)  [unwired: 7 in]
              n441 = call-dynamic "Write Channel.vi"("error in (no error)"=w1204, "Channel.lvclass"=w1206, "Acquisition in"=w1211) -> ("error out"=w1209:errorcluster, "Acquisition out"=w1210:refnum<class "Acquisition.lvclass">)  [unwired: 7 in]
            }
          }
          n442 = call-dynamic "Write AcquisitionC.vi"("error in (no error)"=w1092, "Acquisition.lvclass"=w1093, "S4ACS_GUI in"=w1121) -> ("error out"=w1115:errorcluster, "S4ACS_GUI out"=w1114:refnum<class "S4GUI.lvclass">)  [unwired: 7 in]
          n443 = call-dynamic "Read AcquisitionD.vi"("error in (no error)"=w1115, "S4ACS_GUI in"=w1114) -> ("error out"=w1089:errorcluster, "Acquisition.lvclass"=w1091:refnum<class "Acquisition.lvclass">, "S4ACS_GUI out"=w1120:refnum<class "S4GUI.lvclass">)  [unwired: 7 in]
          n444 = call "Read connection.vi"("error in (no error)"=w1089, "Server in"=w1091) -> ("error out"=w1088:errorcluster, "connection"=w1087:bool, "Server out"=w1090:refnum<class "Acquisition.lvclass">)  [unwired: 7 in]
          n445 = case shown="True" w1087 {
            tunnel: w1090 -> [w1179 w1195]
            tunnel: w1088 -> [w1178 w1194]
            tunnel: [w1179 w1192] -> w1086
            tunnel: [w1178 w1191] -> w1085
            tunnel: [0 ("State") w1181] -> w1077
            frame False {
            }
            frame True {
              n446 = call-dynamic "Read Channel.vi"("error in (no error)"=w1194, "Acquisition in"=w1195) -> ("error out"=w1190:errorcluster, "Channel.lvclass"=w1189:refnum<class "Channel.lvclass">, "Acquisition out"=w1193:refnum<class "Acquisition.lvclass">)  [unwired: 7 in]
              n447 = call-dynamic "Read State Machine.vi"("error in (no error)"=w1190, "Device in"=w1189) -> ("error out"=w1183:errorcluster, "State Machine.lvclass"=w1185:refnum<class "State Machine.lvclass">, "Device out"=w1187:refnum<class "Channel.lvclass">)  [unwired: 7 in]
              n448 = call-dynamic "Read State.vi"("error in (no error)"=w1183, "State Machine in"=w1185) -> ("error out"=w1182:errorcluster, "State"=w1181:i32, "State Machine out"=w1184:refnum<class "State Machine.lvclass">)  [unwired: 7 in]
              n449 = call-dynamic "Write State Machine.vi"("error in (no error)"=w1182, "State Machine.lvclass"=w1184, "Device in"=w1187) -> ("error out"=w1186:errorcluster, "Device out"=w1188:refnum<class "Channel.lvclass">)  [unwired: 7 in]
              n450 = call-dynamic "Write Channel.vi"("error in (no error)"=w1186, "Channel.lvclass"=w1188, "Acquisition in"=w1193) -> ("error out"=w1191:errorcluster, "Acquisition out"=w1192:refnum<class "Acquisition.lvclass">)  [unwired: 7 in]
            }
          }
          n451 = call-dynamic "Write AcquisitionD.vi"("error in (no error)"=w1085, "Acquisition.lvclass"=w1086, "S4ACS_GUI in"=w1120) -> ("error out"=w1071:errorcluster, "S4ACS_GUI out"=w1072:refnum<class "S4GUI.lvclass">)  [unwired: 7 in]
          n452 = Equal?(x=w1081, y=w1080) -> (x = y?=w1067:bool)
          n453 = Equal?(x=w1084, y=w1080) -> (x = y?=w1062:bool)
          n454 = Equal?(x=w1081, y=w1079) -> (x = y?=w1061:bool)
          n455 = Equal?(x=w1084, y=w1079) -> (x = y?=w1063:bool)
          n456 = Equal?(x=w1081, y=w1078) -> (x = y?=w1060:bool)
          n457 = Equal?(x=w1084, y=w1078) -> (x = y?=w1064:bool)
          n458 = Equal?(x=w1081, y=w1077) -> (x = y?=w1066:bool)
          n459 = Equal?(x=w1084, y=w1077) -> (x = y?=w1065:bool)
          n460 = call-dynamic "VerifyAcqIdle.vi"("error in (no error)"=w1071, "S4GUI in"=w1072) -> ("error out"=w1069:errorcluster, "idle"=w1068:bool, "S4GUI out"=w1070:refnum<class "S4GUI.lvclass">)  [unwired: 7 in]
          n461 = Compound Arithmetic op=OR(w1062, w1063, w1064, w1065) -> (w1076:bool)
          n462 = Compound Arithmetic op=OR(w1067, w1061, w1060, w1066) -> (w1075:bool)
          n463 = Build Array(w1076, w1075) -> (w1074:bool[])
          n464 = Boolean Array To Number(Boolean array=w1074) -> (number=w1073:u32)
          n465 = case shown="2" w1073 {
            tunnel: w1070 -> [w1135 w1160 w1173 w1177]
            tunnel: [w1134 w1159 w1172 w1176] -> w1082
            tunnel: w1083 -> [w1136 _ _ _]
            tunnel: w1068 -> [w1132 _ _ _]
            tunnel: w1067 -> [_ _ w1170 _]
            tunnel: w1061 -> [_ _ w1169 _]
            tunnel: w1060 -> [_ _ w1168 _]
            tunnel: w1066 -> [_ _ w1167 _]
            tunnel: w1065 -> [_ w1152 _ _]
            tunnel: w1064 -> [_ w1153 _ _]
            tunnel: w1063 -> [_ w1154 _ _]
            tunnel: w1062 -> [_ w1155 _ _]
            frame 0, Default {
              n466 = local read "time307"() -> (w1130:u32)
              n467 = Tick Count (ms)() -> (millisecond timer value=w1131:u32)
              n468 = Subtract(x=w1131, y=w1130) -> (x-y=w1129:u32)
              n469 = Greater?(x=w1129, y=u32 10000) -> (0:w1127:bool)
              n470 = case shown="False" w1127 {
                tunnel: w1136 -> [w1140 _]
                tunnel: [w1139 u32 1 ("Obs_state")] -> w1133
                tunnel: w1132 -> [w1138 _]
                tunnel: ["" w1145] -> w1126
                frame False {
                  n471 = disable-structure shown="Enabled" {
                    disable-tunnel: [299 ("t") 300] -> w1141
                    frame Disabled {
                    }
                    frame Enabled {
                    }
                  }
                  n472 = Select(t=w1141, s=w1138, f=w1140) -> (s? t:f=w1139:u32)
                }
                frame True {
                  n473 = Concatenate Strings("CHANNEL ERROR " ("string"), ": Not idle. S4GUI:HandleObservationSync.vi state 252." ("Error Msg")) -> (w1145:string)
                }
              }
              n474 = Bundle By Name(cluster=w1135, "Obs_state"=w1133, "Error Msg"=w1126) -> (w1134:refnum<class "S4GUI.lvclass">)
            }
            frame 1 {
              n475 = Build Array(w1155, w1154, w1153, w1152) -> (w1157:bool[])
              n476 = Boolean Array To Number(Boolean array=w1157) -> (number=w1156:u32)
              n477 = Number To Decimal String(number=w1156) -> (decimal integer string=w1150:string)  [unwired: 1 in]
              n478 = Concatenate Strings("CHANNEL ERROR < " ("string"), w1150, ">: Initialization failed. S4GUI:HandleObservationSync.vi state 252." ("Error Msg")) -> (w1149:string)
              n479 = Bundle By Name(cluster=w1160, "Obs_state"=u32 1, "Error Msg"=w1149) -> (w1159:refnum<class "S4GUI.lvclass">)
            }
            frame 2 {
              n480 = Build Array(w1170, w1169, w1168, w1167) -> (w1166:bool[])
              n481 = Boolean Array To Number(Boolean array=w1166) -> (number=w1162:u32)
              n482 = Number To Decimal String(number=w1162) -> (decimal integer string=w1161:string)  [unwired: 1 in]
              n483 = Concatenate Strings("CHANNEL ERROR < " ("string"), w1161, ">:  Invalid Exposition Time. S4GUI:HandleObservationSync.vi state 252." ("Error Msg")) -> (w1164:string)
              n484 = Bundle By Name(cluster=w1173, "Obs_state"=u32 1, "Error Msg"=w1164) -> (w1172:refnum<class "S4GUI.lvclass">)
            }
            frame 3 {
              n485 = Bundle By Name(cluster=w1177, "Obs_state"=u32 1, "Error Msg"="ERROR: Invalid configuration in the channels. S4GUI:HandleObservationSync.vi state 252.") -> (w1176:refnum<class "S4GUI.lvclass">)
            }
          }
        }
        frame 253 {
          # "Sem SyncBox, \ntrigger mode = 0 (internal)\nCom SyncBox\ntrigger mode = 6 (ext. start)"
          n486 = call-dynamic "Read Sync Box.lvclass.vi"("error in (no error)"=w1289, "SPARC4_AC in"=w1288) -> ("error out"=w1291:errorcluster, "Sync Box.lvclass"=w1292:refnum<class "Sync Box.lvclass">, "SPARC4_AC out"=w1287:refnum<class "S4GUI.lvclass">)  [unwired: 7 in]
          n487 = call "Read connection.vi"("error in (no error)"=w1291, "Server in"=w1292) -> ("error out"=w1290:errorcluster, "connection"=w1252:bool)  [unwired: 7 in, 1 out]
          n488 = case shown="True" w1252 {
            tunnel: [u8 6 ("TRIGGER_MODE") u8 0 ("TRIGGER_MODE")] -> w1269
            frame True {
            }
            frame False {
            }
          }
          n489 = call-dynamic "Read AcquisitionA.vi"("error in (no error)"=w1290, "S4ACS_GUI in"=w1287) -> ("error out"=w1274:errorcluster, "Acquisition.lvclass"=w1275:refnum<class "Acquisition.lvclass">, "S4ACS_GUI out"=w1273:refnum<class "S4GUI.lvclass">)  [unwired: 7 in]
          n490 = call-dynamic "Read Channel.vi"("error in (no error)"=w1274, "Acquisition in"=w1275) -> ("error out"=w1257:errorcluster, "Channel.lvclass"=w1256:refnum<class "Channel.lvclass">, "Acquisition out"=w1284:refnum<class "Acquisition.lvclass">)  [unwired: 7 in]
          n491 = call-dynamic "Read Interface.vi"("error in (no error)"=w1257, "Channel in"=w1256) -> ("error out"=w1255:errorcluster, "Interface.lvclass"=w1261:refnum<class "Interface.lvclass">, "Channel out"=w1260:refnum<class "Channel.lvclass">)  [unwired: 7 in]
